vi "2진파일에쓰기.vi"() -> ()   [LabVIEW 2014]
uses:
  <vilib>/Analysis/NI_AALBase.lvlib
panel:
  in  "경로":path
  out "에러 출력":errorcluster
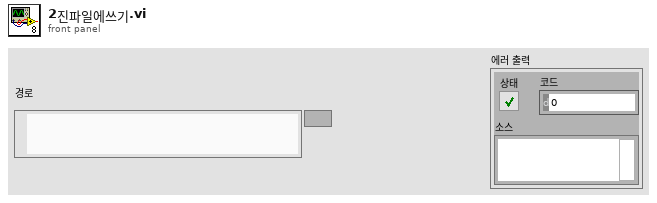
[diagram p1: front panel]
types:
  T1 = enum16{"open", "replace", "create", "open or create", "replace or create", "replace or create with confirmation"}
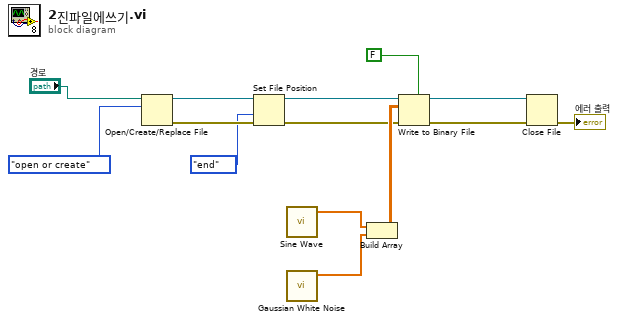
[diagram p0: block diagram]
diagram:
  n1 = Open/Create/Replace File(file path (use dialog)="경로", operation (0:open)=T1."open or create" ("동작(0:open)")) -> (refnum out=w5:refnum<file>, error out=w3:errorcluster)  [unwired: 4 in, 1 out]
  n2 = Set File Position(refnum=w5, from (0:start)=enum16{"start", "end", "current"}."end" ("시작(0:시작)"), error in=w3) -> (refnum out=w4:refnum<file>, error out=w2:errorcluster)  [unwired: 1 in]
  n3 = call <vilib>:"Sine Wave.vi"() -> ("sine wave"=w9:dbl[])  [unwired: 5 in, 2 out]
  n4 = call <vilib>:"Gaussian White Noise.vi"() -> ("Gaussian noise pattern"=w8:dbl[])  [unwired: 10 in, 1 out]
  n5 = Build Array(w9, w8) -> (w7:dbl[][])
  n6 = Write to Binary File(file (use dialog)=w4, data=w7, error in=w2, 5:FALSE ("배열 또는 문자열 크기를 앞에 추가? (참)")) -> (refnum out=w14:refnum<file>, error out=w13:errorcluster)  [unwired: 2 in, 1 out]
  n7 = Close File(refnum=w14, error in=w13) -> (error out=→"에러 출력":errorcluster)  [unwired: 1 out]
